vi "GetTerms3.vi"(0 "XRef":T10, 1 "State In":T9) -> (14 "Terms":T1)   [LabVIEW 2012, in "CThread.lvlib" / "CThread VI Terminal Node.xnode"]
doc: "This ability VI is used to describe your terminals to LabVIEW. Terms is an array of clusters describing the XNode's terminals.\n ID: A unique string identifying the terminal.\n Name: The name of the terminal visible to the user. Remember to localize it.\n Type: The data type of the terminal (as a Variant). The data put in the variant will be used as the default for the input terminal if it's left unwired.\n Bounds: A rectangle defining the bounds of the terminal relative to the bounds of the XNode. The bounds must be within the bounds of the XNode, and for whiskers to draw properly, they must be flush with at least one side of the XNode.\n Input?: Indicates whether or not this terminals is an input.\n Required?: Indicates whether the user must wire this terminal for the XNode to not be broken. Ignored on outputs.\n Recommended?: Indicates whether the terminal is recommended.\n Hidden?: Indicates whether the terminal is hidden. When a terminal is hidden, it cannot be wired to via user interaction or scripting. However, if it is already wired to when the hidden flag is changed to true, it will remain wired.\n Adaptive?: Indicates that the term should change to match the type of its source if it is wired.\n Direction?: Indicates what direction the wire stub should point. Choose auto to let LV decide based on the terms bounds being on the nodes edge.\n \n The IDs are used by LabVIEW to keep track of your terminals. When you respecify your terminals, LabVIEW can tell whther terminals are new, deleted, or moved by the unique IDs. The order is irrelevant. If you move a terminal, then any wire connected to it will move with it.\n \n If you want to update your terminals, you should return the UpdateTerms reply in one of your ability VIs.\n\nDefault behavior: None.\n\nThis ability does not provide UI and OS messages are not handled."
uses:
  CThread VI Terminal Node.xnode
  <vilib>/XNodeSupport/XNodeXNodeRef.ctl
  State.ctl
  <vilib>/XNodeSupport/XNodeTerm3Array.ctl
  <vilib>/XNodeSupport/XNodeTerm3.ctl
  <vilib>/XNodeSupport/XNodeString.ctl
  <vilib>/XNodeSupport/XNodeVariant.ctl
  <vilib>/XNodeSupport/XNodeRect32.ctl
  <vilib>/XNodeSupport/XNodeInt.ctl
  <vilib>/XNodeSupport/XNodeBool.ctl
  <vilib>/XNodeSupport/XNodeTermDirection.ctl
  <vilib>/XNodeSupport/NI_XNodeSupport.lvlib
panel:
  in  "CLIB VI Reference":i32
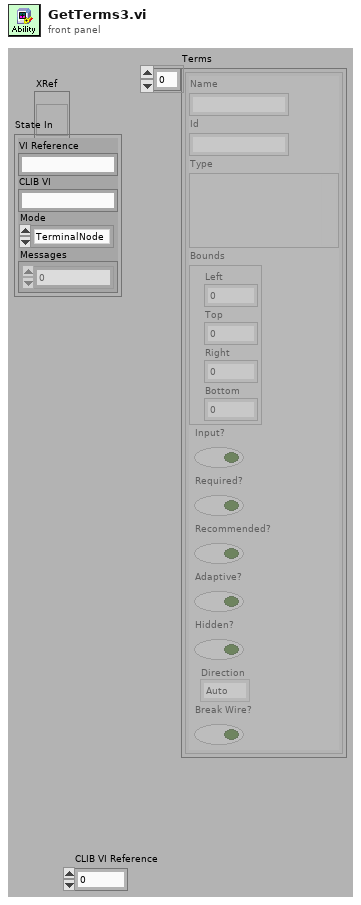
[diagram p1: front panel]
types:
  T1 = typedef "NI_XNodeSupport.lvlib/XNodeTerm3Array.ctl" = T2[]
  T2 = typedef "NI_XNodeSupport.lvlib/XNodeTerm3.ctl" = cluster{"Name":T3, "Id":T3, "Type":T4, "Bounds":T5, "Input?":T7, "Required?":T7, "Recommended?":T7, "Adaptive?":T7, "Hidden?":T7, "Direction":T8, "Break Wire?":T7}
  T3 = typedef "NI_XNodeSupport.lvlib/XNodeString.ctl" = string
  T4 = typedef "NI_XNodeSupport.lvlib/XNodeVariant.ctl" = variant
  T5 = typedef "NI_XNodeSupport.lvlib/XNodeRect32.ctl" = cluster{"Left":T6, "Top":T6, "Right":T6, "Bottom":T6}
  T6 = typedef "NI_XNodeSupport.lvlib/XNodeInt.ctl" = i32
  T7 = typedef "NI_XNodeSupport.lvlib/XNodeBool.ctl" = bool
  T8 = typedef "NI_XNodeSupport.lvlib/XNodeTermDirection.ctl" = enum32{"Auto", "Up", "Down", "Left", "Right", "Center"}
  T9 = typedef "CThread.lvlib/CThread VI Terminal Node.xnode/State.ctl" = cluster{"VI Reference":string, "CLIB VI":string, "Mode":enum16{"TerminalNode", "AdaptorNode"}, "Messages":u8[]}
  T10 = typedef "NI_XNodeSupport.lvlib/XNodeXNodeRef.ctl" = refnum<vi>
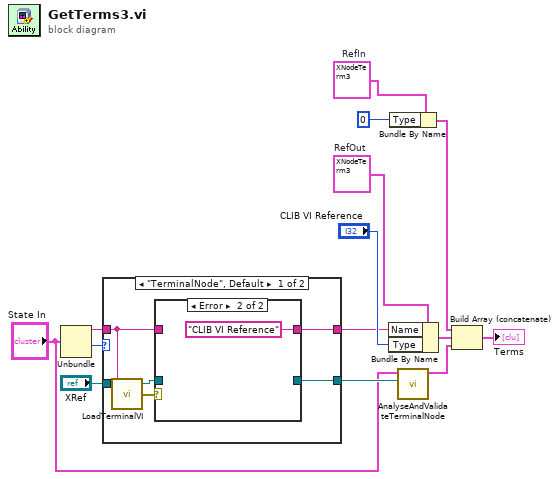
[diagram p0: block diagram]
diagram:
  w14 = T2 {"Name"="CLIB VI Reference", "Id"="RefIn", "Type"=variant, "Bounds"={"Left"=0, "Top"=0, "Right"=15, "Bottom"=8}, "Input?"=TRUE, "Required?"=TRUE, "Recommended?"=FALSE, "Adaptive?"=FALSE, "Hidden?"=FALSE, "Direction"=enum."Left", "Break Wire?"=FALSE}  # RefIn
  w13 = T2 {"Name"="CLIB VI Reference", "Id"="RefOut", "Type"=variant, "Bounds"={"Left"=16, "Top"=0, "Right"=32, "Bottom"=8}, "Input?"=FALSE, "Required?"=FALSE, "Recommended?"=FALSE, "Adaptive?"=FALSE, "Hidden?"=FALSE, "Direction"=enum."Right", "Break Wire?"=FALSE}  # RefOut
  n1 = Unbundle("State In") -> ("VI Reference"=w7:string, "Mode"=w6:enum16{"TerminalNode", "AdaptorNode"})  [unwired: 2 out]
  n2 = case shown="\"TerminalNode\", Default" w6 {
    tunnel: [w20 w24] -> w8
    tunnel: w7 -> [w15 w24]
    tunnel: [w19 _] -> w4
    tunnel: "XRef" -> [w16 _]
    frame "TerminalNode", Default {
      n3 = call "LoadTerminalVI.vi"("VI Reference"=w15, "XRef"=w16) -> ("error out"=w17:errorcluster, "vi reference"=w18:refnum<vi>)  [unwired: 2 in]
      n4 = case shown="Error" w17 {
        tunnel: w18 -> [w21 _]
        tunnel: w15 -> [w22 _]
        tunnel: [w22 "CLIB VI Reference" ("VI")] -> w20
        tunnel: [w21 _] -> w19
        frame No Error {
        }
        frame Error {
        }
      }
    }
    frame "AdaptorNode" {
    }
  }
  n5 = Bundle By Name(cluster=w13, "Name"=w8, "Type"="CLIB VI Reference") -> (w11:T2)
  n6 = Bundle By Name(cluster=w14, "Type"=0 ("BoundsOffset-Y")) -> (w12:T2)
  n7 = call "AnalyseAndValidateTerminalNode.vi"("Comparison VI"=w4, "State"="State In") -> ("Terms"=w3:T2[])  [unwired: 6 in, 3 out]
  n8 = Build Array (concatenate)(w12, w11, w3) -> (→"Terms":T2[])
